vi "Error Query (Multiple).vi"(0 "VISA Resource Name":refnum<visa-resource-name>, 11 "error in (no error)":errorcluster) -> (4 "VISA Resource Name Out":refnum<visa-resource-name>, 8 "Error":i32[](array[numeric]), 10 "Error Message":string, 15 "error out":errorcluster)   [LabVIEW 2012, in "Agilent 34970.lvlib"]
doc: "This VI reads the error queue from the instrument. It expects to see errors in SCPI format (#,\"error message\"). It continues to read from the error queue until it reads a 0, \"No error\". If the instrument does not support an error query, a warning is returned."
uses:
  <instrlib>/Agilent 34970/Agilent 34970.lvlib
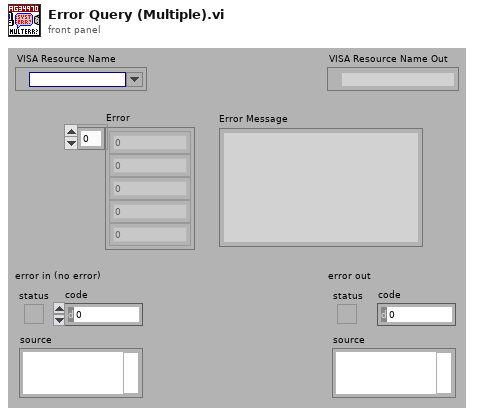
[diagram p1: front panel]
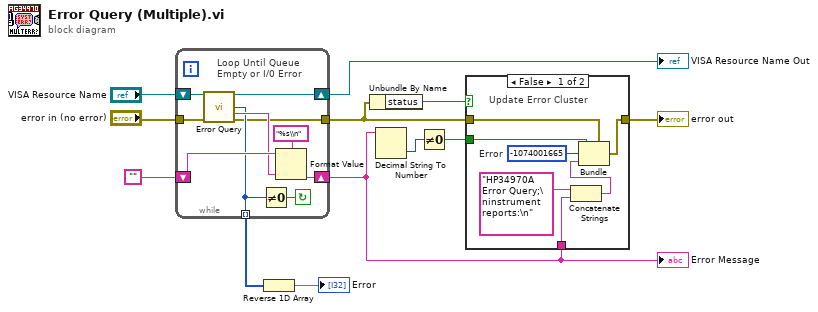
[diagram p0: block diagram]
diagram:
  n1 = while {
    tunnel: "error in (no error)" -> [w13]
    tunnel: [w16] -> w6 mode=indexing
    tunnel: [w14] -> w9
    shift-left: "VISA Resource Name" -> [w15]
    shift-right: [w22] -> w5
    shift-left: "" ("Empty String Constant") -> [w19]
    shift-right: [w21] -> w11
    stop <- w17 continue-if-true
    # "Loop Until Queue Empty or I/0 Error"
    n2 = call <instrlib>:"Error Query.vi"("VISA Resource Name"=w15, "error in (no error)"=w13) -> ("VISA Resource Name Out"=w22:refnum<visa-resource-name>, "Error"=w16:i32, "Error Message"=w18:string, "error out"=w14:errorcluster)  [unwired: 10 in]
    n3 = Not Equal To 0?(x=w16) -> (x != 0?=w17:bool)
    n4 = Format Value(string ("")=w19, format string="%s\\n", value (0)=w18) -> (output string=w21:string)
  }
  "Error Message" <- w11
  "VISA Resource Name Out" <- w5
  n5 = Reverse 1D Array(array=w6) -> (reversed array=→"Error":i32[])
  n6 = Unbundle By Name(w9) -> ("status"=w8:bool)
  n7 = Decimal String To Number(string=w11) -> (number=w10:i32)  [unwired: 2 in, 1 out]
  n8 = Not Equal To 0?(x=w10) -> (x != 0?=w7:bool)
  n9 = case shown="False" w8 {
    tunnel: w9 -> [w28 w30]
    tunnel: [w27 w30] -> w4
    tunnel: w11 -> [w24 _]
    tunnel: w7 -> [w23 _]
    frame False {
      w29 = -1074001665  # Error
      # "Update Error Cluster"
      n10 = Concatenate Strings("HP34970A Error Query;\ninstrument reports:\n", w24) -> (w26:string)
      n11 = Bundle(cluster=w28, "status"=w23, "code"=w29, "source"=w26) -> (w27:errorcluster)
    }
    frame True {
      # "No Instrument Errors"
    }
  }
  "error out" <- w4
